vi "TfidfTransformer.vi"(8 "error in":errorcluster caption="entrée d'erreur", 11 "TfidfTransformer":T1={"norm"="l2", "use_idf"=TRUE, "smooth_idf"=TRUE, "sublinear_tf"=FALSE}) -> (0 "error out":errorcluster caption="sortie d'erreur", 3 "TfidfTransformer.lvclass":refnum<class "TfidfTransformer.lvclass">)   [LabVIEW 2020]
doc: "Transform a count matrix to a normalized tf or tf-idf representation\n\nTf means term-frequency while tf-idf means term-frequency times inverse document-frequency. This is a common term weighting scheme in information retrieval, that has also found good use in document classification.\n\nThe goal of using tf-idf instead of the raw frequencies of occurrence of a token in a given document is to scale down the impact of tokens that occur very frequently in a given corpus and that are hence empirically less informative than features that occur in a small fraction of the training corpus.\n\nThe formula that is used to compute the tf-idf for a term t of a document d in a document set is tf-idf(t, d) = tf(t, d) * idf(t), and the idf is computed as idf(t) = log [ n / df(t) ] + 1 (if smooth_idf=False), where n is the total number of documents in the document set and df(t) is the document frequency of t; the document frequency is the number of documents in the document set that contain the term t. The effect of adding “1” to the idf in the equation above is that terms with zero idf, i.e., terms that occur in all documents in a training set, will not be entirely ignored. (Note that the idf formula above differs from the standard textbook notation that defines the idf as idf(t) = log [ n / (df(t) + 1) ]).\n\nIf smooth_idf=True (the default), the constant “1” is added to the numerator and denominator of the idf as if an extra document was seen containing every term in the collection exactly once, which prevents zero divisions: idf(t) = log [ (1 + n) / (1 + df(t)) ] + 1.\n\nFurthermore, the formulas used to compute tf and idf depend on parameter settings that correspond to the SMART notation used in IR as follows:\n\nTf is “n” (natural) by default, “l” (logarithmic) when sublinear_tf=True. Idf is “t” when use_idf is given, “n” (none) otherwise. Normalization is “c” (cosine) when norm='l2', “n” (none) when norm=None.\n\n\nParameters : \n\n- norm : {‘l1’, ‘l2’}, default=’l2’\nEach output row will have unit norm, either: * ‘l2’: Sum of squares of vector elements is 1. The cosine similarity between two vectors is their dot product when l2 norm has been applied. * ‘l1’: Sum of absolute values of vector elements is 1. See preprocessing.normalize\n\n- use_idf : bool, default=True\nEnable inverse-document-frequency reweighting.\n\n- smooth_idf : bool, default=True\nSmooth idf weights by adding one to document frequencies, as if an extra document was seen containing every term in the collection exactly once. Prevents zero divisions.\n\n- sublinear_tf : bool, default=False\nApply sublinear tf scaling, i.e. replace tf with 1 + log(tf).\n\n\nMethods : \n\n\n- Fit : Learn the idf vector (global term weights).\n\nParameters : X : sparse matrix of shape n_samples, n_features)\n A matrix of term/token counts.\n\n\n- Fit Transform : Fit to data, then transform it. Fits transformer to X and y with optional parameters fit_params and returns a transformed version of X.\n\nParameters : X : {array-like, sparse matrix, dataframe} of shape (n_samples, n_features)\n y : ndarray of shape (n_samples,), default=None\n Target values.\n\nReturns : X_new : ndarray array of shape (n_samples, n_features_new)\n Transformed array.\n\n- Transform : Transform a count matrix to a tf or tf-idf representation\n\nParameters : X : sparse matrix of (n_samples, n_features)\n a matrix of term/token counts\n\nReturns : vectors : sparse matrix of shape (n_samples, n_features)"
uses:
  TfidfTransformer.lvclass
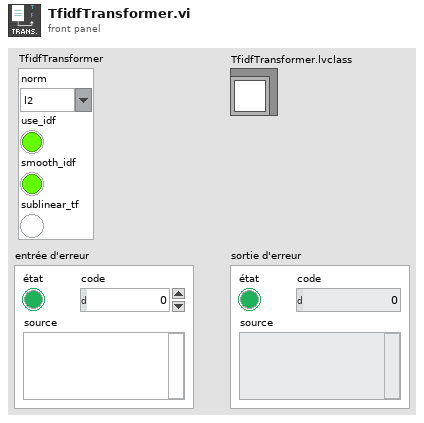
[diagram p1: front panel]
types:
  T1 = cluster{"norm":string, "use_idf":bool, "smooth_idf":bool, "sublinear_tf":bool}
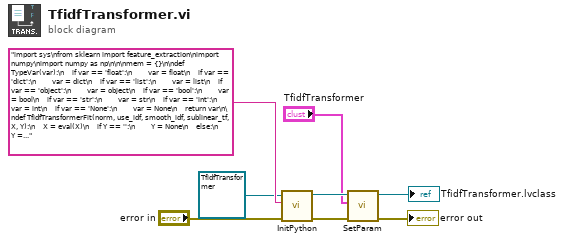
[diagram p0: block diagram]
diagram:
  n1 = call-dynamic "InitPython.vi"("error in (no error)"="error in", "Python Instruction"="import sys\nfrom sklearn import feature_extraction\nimport numpy\nimport numpy as np\n\n\nmem = {}\n\ndef TypeVar(var):\n    if var == 'float':\n        var = float\n    if var == 'dict':\n        var = dict\n    if var == 'list':\n        var = list\n    if var == 'object':\n        var = object\n    if var == 'bool':\n        var = bool\n    if var == 'str':\n        var = str\n    if var == 'int':\n        var = int\n    if var == 'None':\n        var = None\n    return var\n\ndef TfidfTransformerFit(norm, use_idf, smooth_idf, sublinear_tf, X, Y):\n    X = eval(X)\n    if Y == '':\n        Y = None\n    else:\n        Y = eval(Y)\n    try:\n        TfidfTransformer = feature_extraction.text.TfidfTransformer(norm, use_idf, smooth_idf, sublinear_tf).fit(X, Y)\n        mem['FitTfidfTransformer'] = TfidfTransformer\n        return str('OK')\n    except:\n        erreur = sys.exc_info()\n        typerr = u\"%s\" % (erreur[0])\n        typerr = typerr[typerr.find(\"'\")+1:typerr.rfind(\"'\")]\n        msgerr = u\"%s\" % (erreur[1])\n        message = str('/!\\\\ {0} : {1}'. format(typerr,msgerr))\n        return message \n\ndef TfidfTransformerFitTransform(norm, use_idf, smooth_idf, sublinear_tf, X, Y):\n    X = eval(X)\n    if Y == '':\n        Y = None\n    else:\n        Y = eval(Y)\n    try:\n        TfidfTransformer = feature_extraction.text.TfidfTransformer(norm, use_idf, smooth_idf, sublinear_tf).fit_transform(X, Y)\n        dtype = type(TfidfTransformer)\n        if dtype == numpy.ndarray:\n            TfidfTransformer = TfidfTransformer.tolist()\n            return str(TfidfTransformer)\n        else:\n            Mat = TfidfTransformer.tocoo()\n            return str(list(zip(Mat.row, Mat.col, Mat.data)))\n    except:\n        erreur = sys.exc_info()\n        typerr = u\"%s\" % (erreur[0])\n        typerr = typerr[typerr.find(\"'\")+1:typerr.rfind(\"'\")]\n        msgerr = u\"%s\" % (erreur[1])\n        message = str('/!\\\\ {0} : {1}'. format(typerr,msgerr))\n        return message \n    \ndef TfidfTransformerTransform(norm, use_idf, smooth_idf, sublinear_tf, X, Y):\n    X = eval(X)\n    if Y == '':\n        Y = None\n    else:\n        Y = eval(Y)\n    try:\n        TfidfTransformer = mem['FitTfidfTransformer'].transform(X, Y)\n        dtype = type(TfidfTransformer)\n        if dtype == numpy.ndarray:\n            TfidfTransformer = TfidfTransformer.tolist()\n            return str(TfidfTransformer)\n        else:\n            Mat = TfidfTransformer.tocoo()\n            return str(list(zip(Mat.row, Mat.col, Mat.data)))\n    except:\n        erreur = sys.exc_info()\n        typerr = u\"%s\" % (erreur[0])\n        typerr = typerr[typerr.find(\"'\")+1:typerr.rfind(\"'\")]\n        msgerr = u\"%s\" % (erreur[1])\n        message = str('/!\\\\ {0} : {1}'. format(typerr,msgerr))\n        return message", "Scikit-learn en entrée"=refnum<class "TfidfTransformer.lvclass"> refnum ("TfidfTransformer.lvclass")) -> ("error out"=w5:errorcluster, "Scikit-learn en sortie"=w4:refnum<class "TfidfTransformer.lvclass">)  [unwired: 7 in]
  n2 = call-dynamic "SetParam.vi"("error in (no error)"=w5, "TfidfTransformer"="TfidfTransformer", "TfidfTransformer.lvclass"=w4) -> ("error out"=→"error out":errorcluster, "TfidfTransformer.lvclass"=→"TfidfTransformer.lvclass":refnum<class "TfidfTransformer.lvclass">)  [unwired: 7 in]
